vi "数据显示.vi"() -> ()   [LabVIEW 2012]
uses:
  <vilib>/Utility/file.llb/Read From Spreadsheet File (DBL).vi
panel:
  out "信号频谱":cluster{dbl, "df":dbl, dbl[]}(graph)
  in  "SAMPLERATE":dbl=512.0 format="%.2f"
  out "信号时间历程":cluster{dbl, "df":dbl, dbl[]}(graph)
  in  "禁用的索引 (列)":i32
  in  "file path (dialog if empty)":path caption="文件路径 （空时为对话框）"
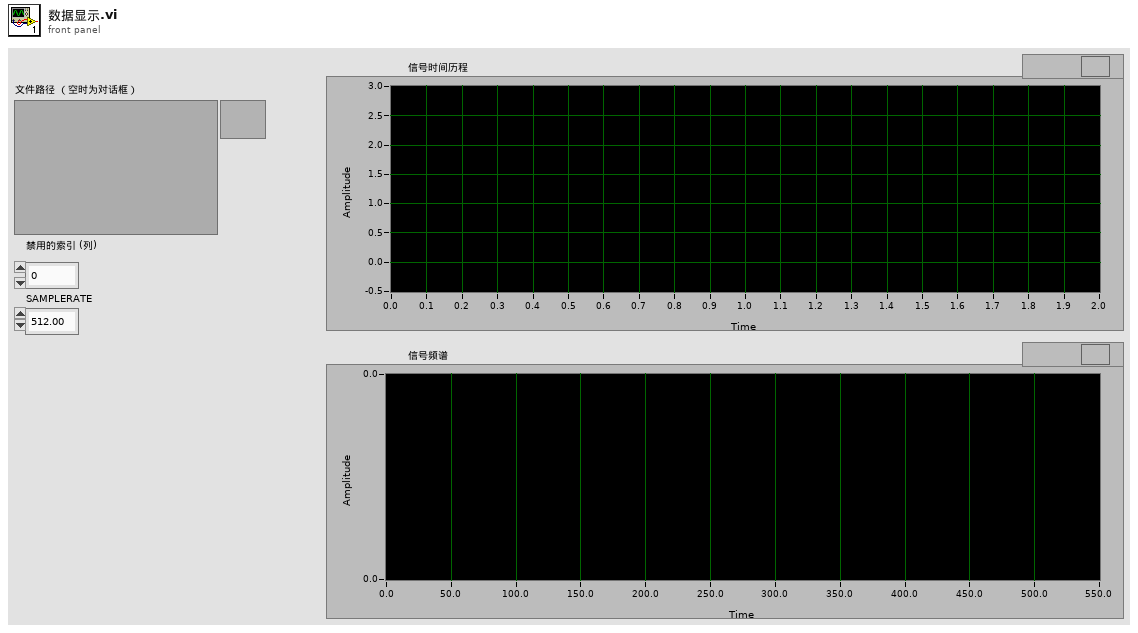
[diagram p1: front panel]
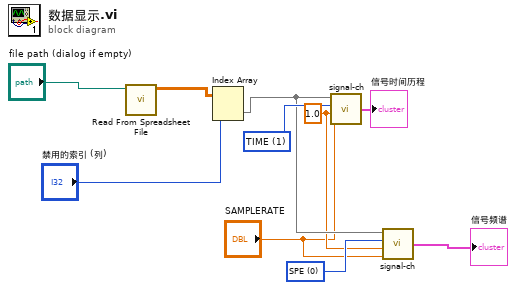
[diagram p0: block diagram]
diagram:
  w4 = u16 0 items=["SPE", "TIME"] ("T/F")
  w3 = 1.0 ("rate")
  w7 = u16 1 items=["SPE", "TIME"] ("T/F")
  n1 = call-poly <vilib>:"Read From Spreadsheet File.vi"("file path (dialog if empty)"="file path (dialog if empty)") -> ("all rows"=w9:dbl[][])  [unwired: 6 in, 4 out]
  n2 = Index Array(array=w9, index (col)="禁用的索引 (列)") -> (element=w5:dbl[])  [unwired: 1 in]
  n3 = call "signal-ch.vi"("sourse"=w5, "T/F"=w7, "rate"=w3, "SAMPLERATE"="SAMPLERATE") -> ("Output Cluster"=→"信号时间历程":cluster{dbl, "df":dbl, dbl[]})  [unwired: 1 in]
  n4 = call "signal-ch.vi"("sourse"=w5, "T/F"=w4, "rate"=w3, "SAMPLERATE"="SAMPLERATE") -> ("Output Cluster"=→"信号频谱":cluster{dbl, "df":dbl, dbl[]})  [unwired: 1 in]
